vi "WLAN_be_EVM_SA_RS_CMP180.vi"(6 "SG Power":i32=-10, 7 "Function":T1, 8 "error in":errorcluster, 11 "VISA IN":refnum<visa-resource-name>="TCPIP0::192.168.200.50::hislip0::INSTR") -> (0 "error out":errorcluster, 1 "EVM":dbl format="%#.3g", 2 "Power":dbl format="%#.3g", 3 "IDN":string, 4 "FreqError":dbl)   [LabVIEW 2023, in "R_S.lvlib"]
uses:
  R_S.lvlib
  CTL/LitePoint_EVM_SA.ctl
panel:
  out "SecondTime":i32
  out "FirstTime":i32
  in  "Retry Times":i32=100
  out "Response":string
  out "String":string
  out "EVM_ALL_Carrier_Mean":string
  out "PPDU_Power_Mean":string
  out "VSA?":string
  # "CMP180: TCPIP0::192.168.200.50::hislip0::INSTR"
  # "TCPIP::Vince_Wu-NB::inst0::INSTR"
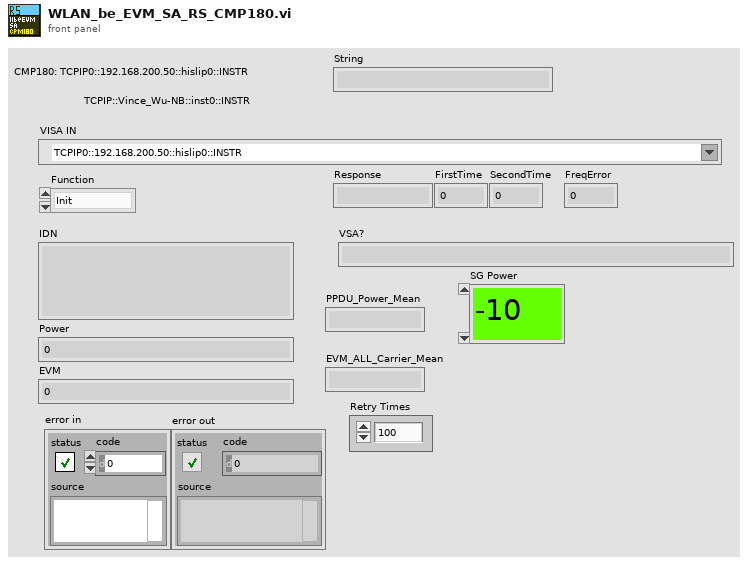
[diagram p1: front panel]
types:
  T1 = typedef "LitePoint_EVM_SA.ctl" = enum16{"Init", "Close", "set_SA", "get_EVM", "byPass", "getPower"}
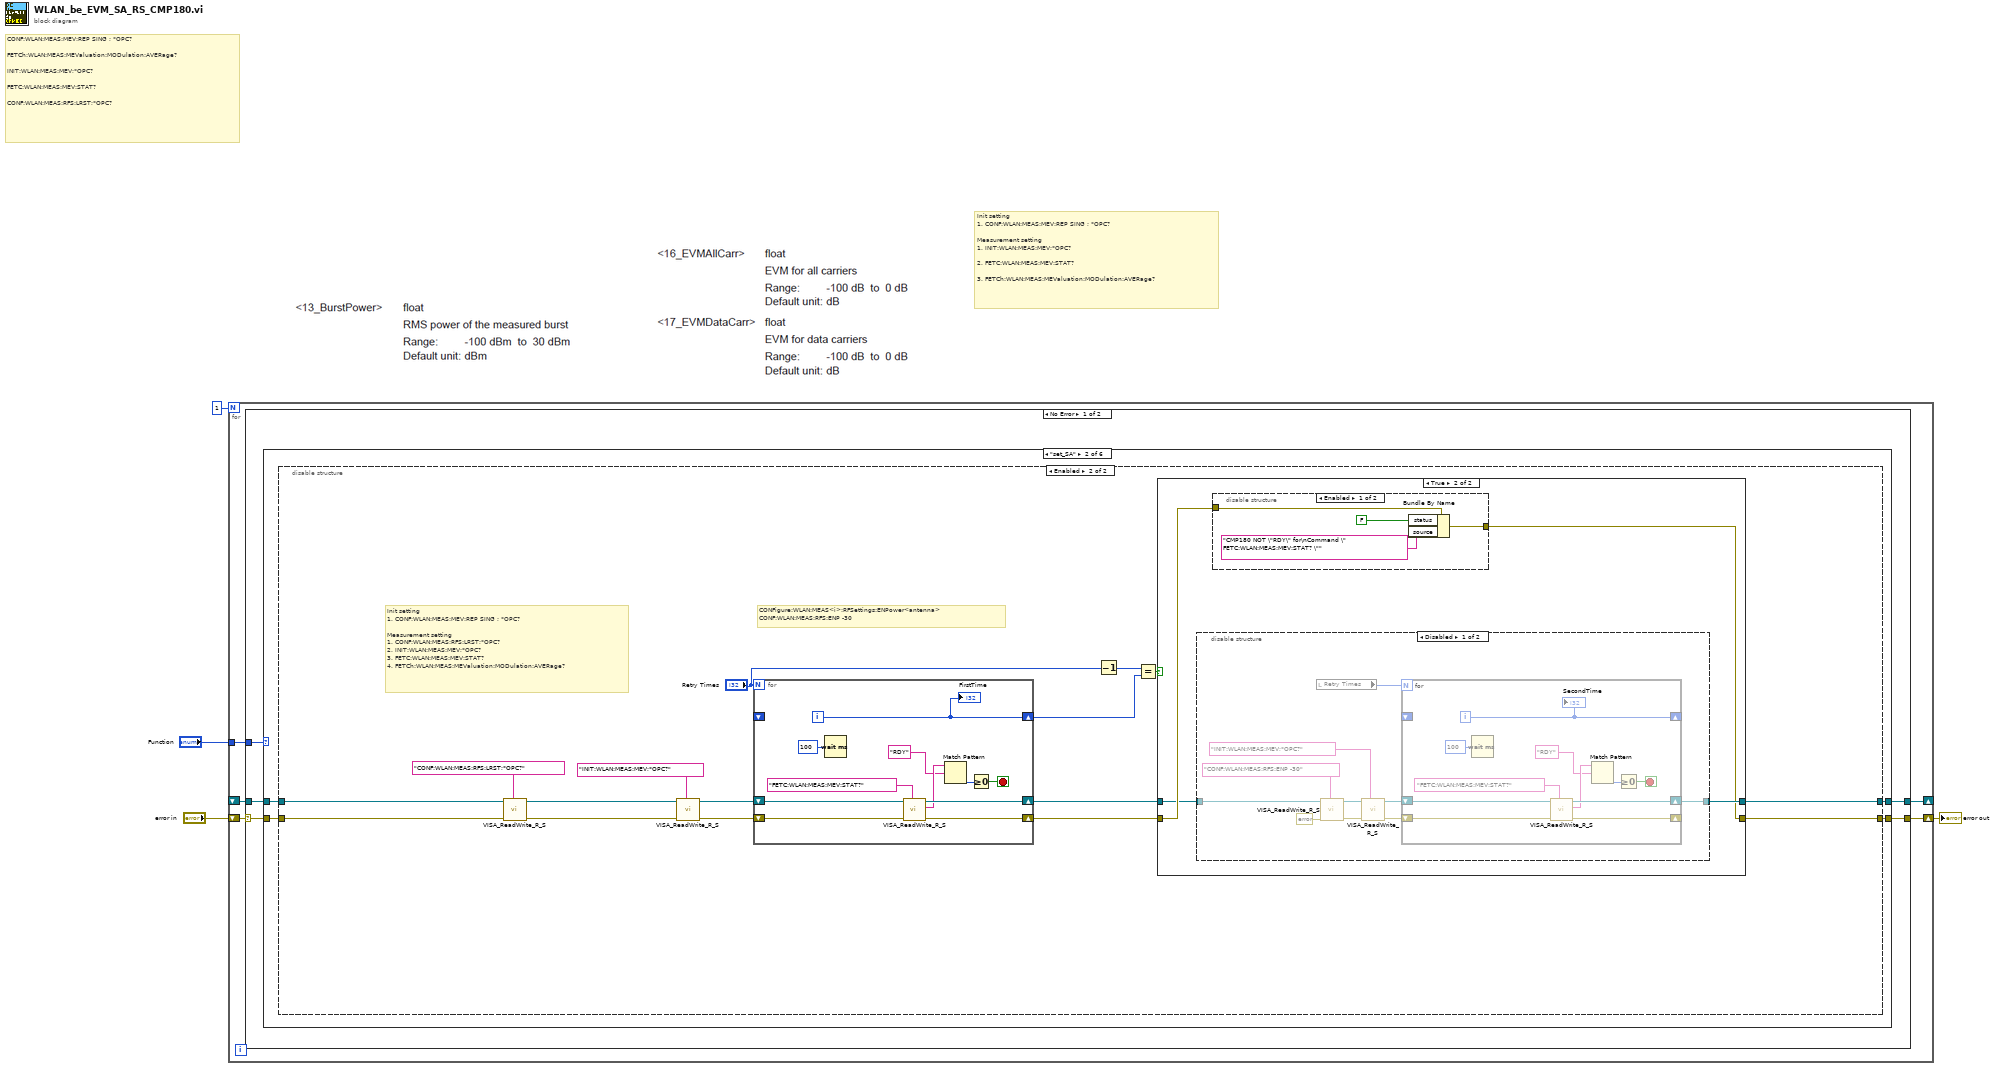
[diagram p0: block diagram]
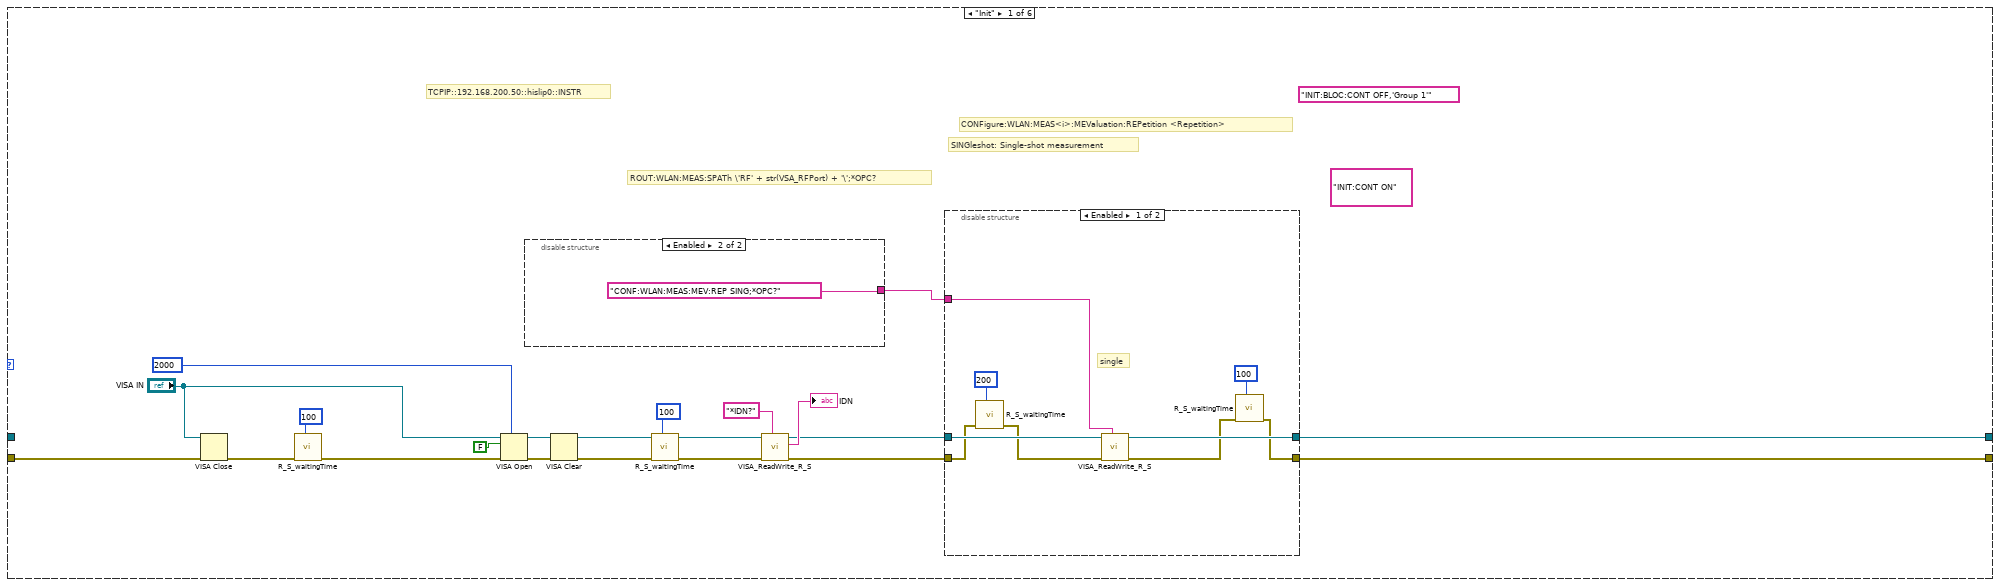
[diagram p2: hidden frame]
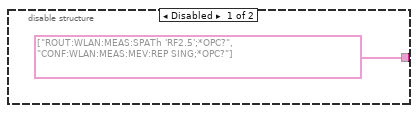
[diagram p3: hidden frame]
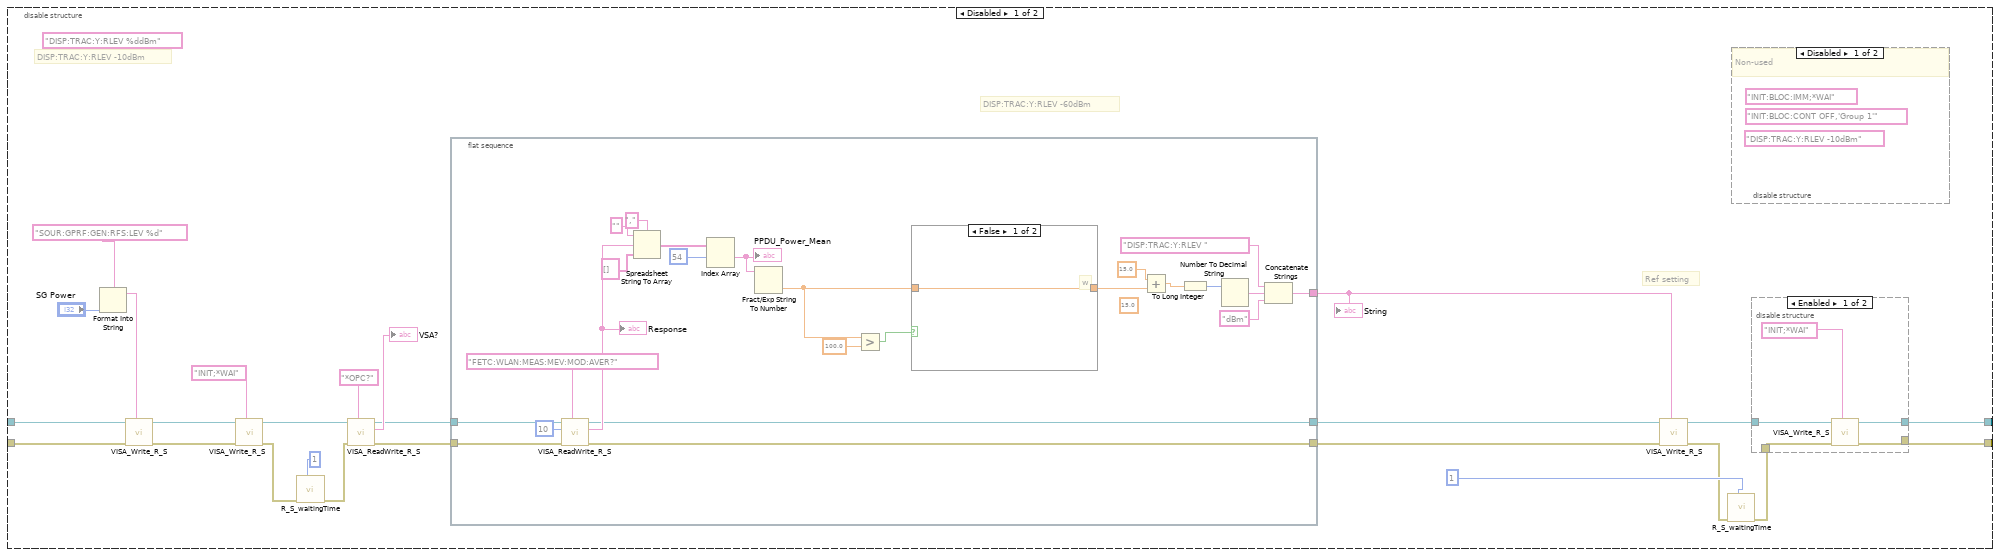
[diagram p5: hidden frame]
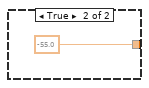
[diagram p7: hidden frame]
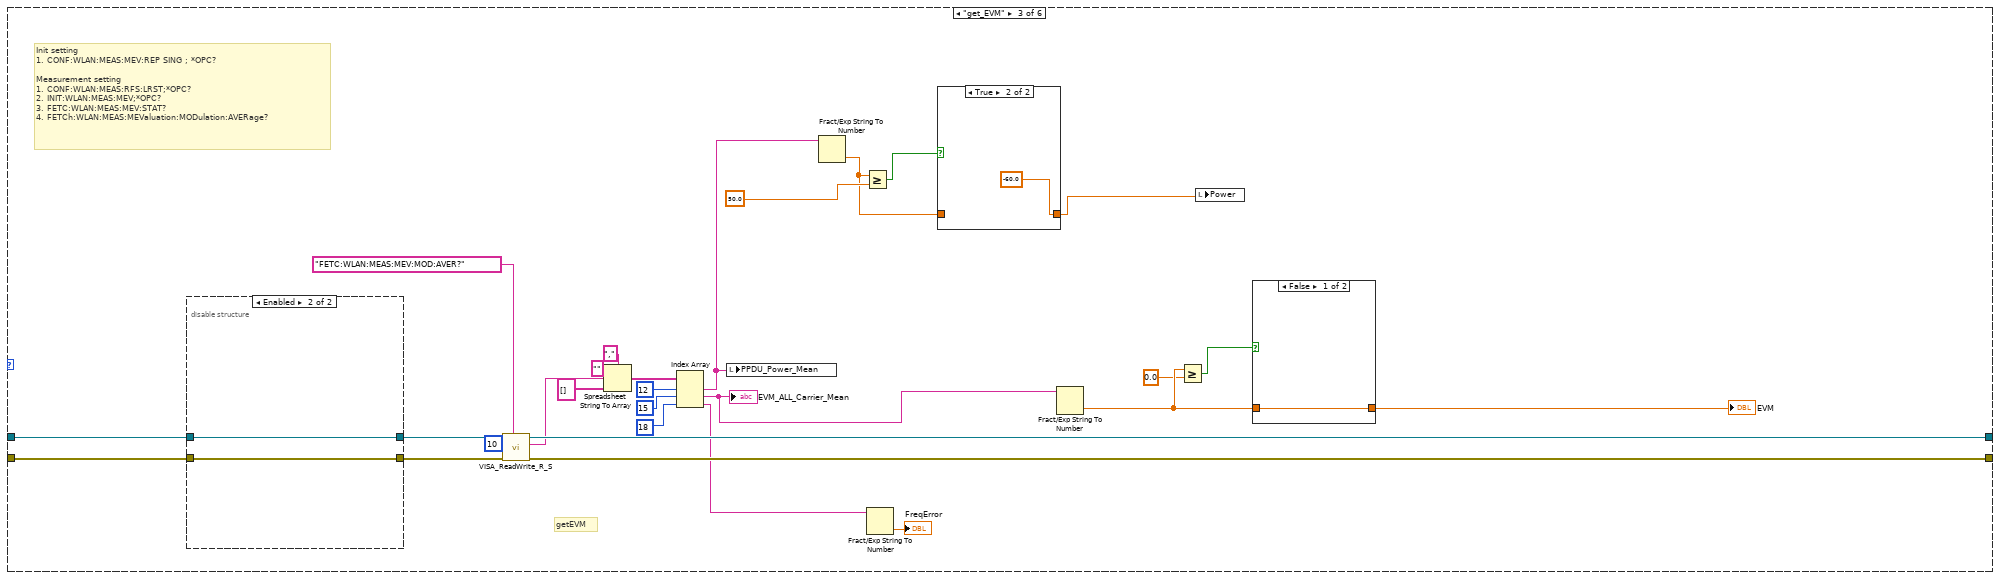
[diagram p12: hidden frame]
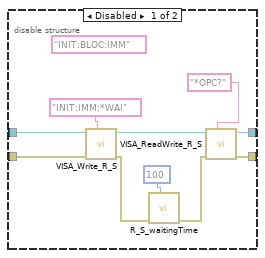
[diagram p13: hidden frame]
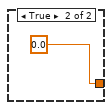
[diagram p15: hidden frame]
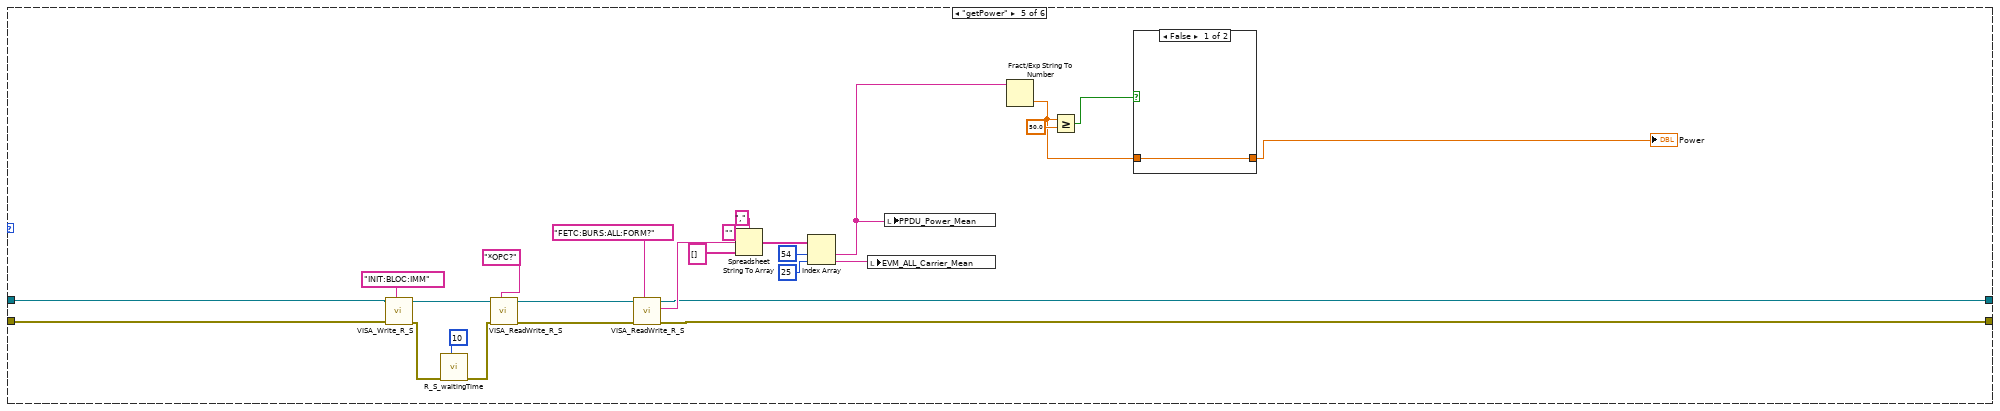
[diagram p17: hidden frame]
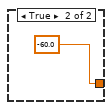
[diagram p18: hidden frame]
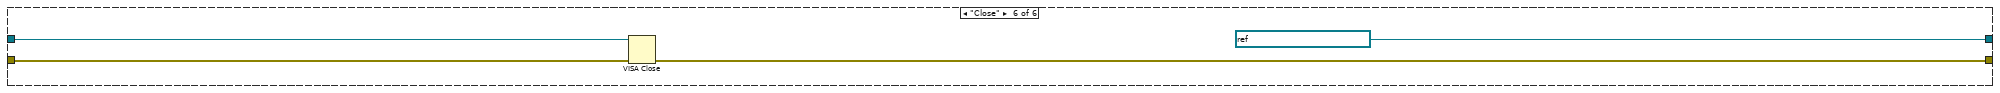
[diagram p19: hidden frame]
diagram:
  # "Init setting\n1. CONF:WLAN:MEAS:MEV:REP SING ; *OPC?\n\nMeasurement setting\n1. INIT:WLAN:MEAS:MEV;*OPC?\n\n2. FETC:WLAN:MEAS:MEV:STAT?\n\n3. FETCh:WLAN:MEAS:MEValuation:MODulation:AVERage?"
  # "CONF:WLAN:MEAS:MEV:REP SING ; *OPC?\n\nFETCh:WLAN:MEAS:MEValuation:MODulation:AVERage?\n\nINIT:WLAN:MEAS:MEV;*OPC?\n\nFETC:WLAN:MEAS:MEV:STAT?\n\nCONF:WLAN:MEAS:RFS:LRST;*OPC?"
  n1 = for {
    N: 1 -> [_]
    tunnel: "Function" -> [w7]
    shift-right: [w8] -> w3
    shift-left: "error in" -> [w9]
    shift-right: [w5] -> _
    shift-left: _ -> [w6]
    n2 = case shown="No Error" w9 {
      selector: w9 -> [w13 w249]
      tunnel: [w12 w249] -> w8
      tunnel: w7 -> [w14 _]
      tunnel: w6 -> [w11 w248]
      tunnel: [w10 w248] -> w5
      frame No Error {
        n3 = case shown="\"set_SA\"" w14 {
          tunnel: [w24 w51 w189 w215 w219 w247] -> w12
          tunnel: w13 -> [w27 w49 w190 w215 w221 w246]
          tunnel: w11 -> [_ w48 w188 w214 w222 w245]
          tunnel: [w22 w50 w187 w214 w220 refnum<visa-resource-name> refnum ("VISA out")] -> w10
          frame "Init" {
            (unwired) "INIT:BLOC:CONT OFF,'Group 1'"
            (unwired) "INIT:CONT ON"
            # "ROUT:WLAN:MEAS:SPATh \\'RF' + str(VSA_RFPort) + '\\';*OPC?"
            # "TCPIP::192.168.200.50::hislip0::INSTR"
            # "SINGleshot: Single-shot measurement"
            # "CONFigure:WLAN:MEAS<i>:MEValuation:REPetition <Repetition>"
            n4 = VISA Close(VISA resource name="VISA IN", error in (no error)=w27) -> (error out=w21:errorcluster)
            n5 = call "R_S_waitingTime.vi"("Waiting Time(ms)"=u32 100, "error in"=w21) -> ("error out"=w20:errorcluster)  [unwired: 9 in]
            n6 = VISA Open(timeout (0)=u32 2000 ("VISA Open timeout (0)"), duplicate session (F)=FALSE, error in (no error)=w20, VISA resource name="VISA IN") -> (VISA resource name=w31:refnum<visa-resource-name>, error out=w32:errorcluster)  [unwired: 1 in]
            n7 = disable-structure shown="Enabled" {
              disable-tunnel: [string[] ["ROUT:WLAN:MEAS:SPATh 'RF2.5';*OPC?", "CONF:WLAN:MEAS:MEV:REP SING;*OPC?"] "CONF:WLAN:MEAS:MEV:REP SING;*OPC?"] -> w15
              frame Disabled {
              }
              frame Enabled {
              }
            }
            n8 = VISA Clear(VISA resource name=w31, error in (no error)=w32) -> (VISA resource name out=w30:refnum<visa-resource-name>, error out=w17:errorcluster)
            n9 = call "R_S_waitingTime.vi"("Waiting Time(ms)"=u32 100, "error in"=w17) -> ("error out"=w16:errorcluster)  [unwired: 9 in]
            n10 = call "VISA_ReadWrite_R_S.vi"("VISA_CMD"="*IDN?", "error in"=w16, "VISA in"=w30) -> ("error out"=w25:errorcluster, "Response"=→"IDN":string, "VISA out"=w23:refnum<visa-resource-name>)  [unwired: 6 in]
            n11 = disable-structure shown="Enabled" {
              disable-tunnel: w25 -> [w41 w47]
              disable-tunnel: [w38 w47] -> w24
              disable-tunnel: w23 -> [w45 w46]
              disable-tunnel: [w44 w46] -> w22
              disable-tunnel: w15 -> [w37 _]
              frame Enabled {
                # "single"
                n12 = call "R_S_waitingTime.vi"("Waiting Time(ms)"=u32 200, "error in"=w41) -> ("error out"=w42:errorcluster)  [unwired: 9 in]
                n13 = call "VISA_ReadWrite_R_S.vi"("VISA_CMD"=w37, "error in"=w42, "VISA in"=w45) -> ("error out"=w39:errorcluster, "VISA out"=w44:refnum<visa-resource-name>)  [unwired: 6 in, 1 out]
                n14 = call "R_S_waitingTime.vi"("Waiting Time(ms)"=u32 100, "error in"=w39) -> ("error out"=w38:errorcluster)  [unwired: 9 in]
              }
              frame Disabled {
              }
            }
          }
          frame "set_SA" {
            n15 = disable-structure shown="Enabled" {
              disable-tunnel: [w63 w117] -> w51
              disable-tunnel: [w62 w115] -> w50
              disable-tunnel: w49 -> [w59 w111]
              disable-tunnel: w48 -> [w58 w110]
              frame Disabled {
                (unwired) "DISP:TRAC:Y:RLEV %ddBm" ("VISA CMD")
                # "DISP:TRAC:Y:RLEV -10dBm"
                # "Ref setting"
                # "DISP:TRAC:Y:RLEV -60dBm"
                n16 = Format Into String(format string="SOUR:GPRF:GEN:RFS:LEV %d" ("VISA CMD"), "SG Power") -> (resulting string=w52:string)  [unwired: 2 in, 1 out]
                n17 = call "VISA_Write_R_S.vi"("VISA CMD"=w52, "error in"=w59, "VISA in"=w58) -> ("error out"=w55:errorcluster, "VISA out"=w56:refnum<visa-resource-name>)  [unwired: 7 in]
                n18 = call "VISA_Write_R_S.vi"("VISA CMD"="INIT;*WAI", "error in"=w55, "VISA in"=w56) -> ("error out"=w61:errorcluster, "VISA out"=w60:refnum<visa-resource-name>)  [unwired: 7 in]
                n19 = call "R_S_waitingTime.vi"("Waiting Time(ms)"=u32 1, "error in"=w61) -> ("error out"=w76:errorcluster)  [unwired: 9 in]
                n20 = call "VISA_ReadWrite_R_S.vi"("VISA_CMD"="*OPC?", "error in"=w76, "VISA in"=w60) -> ("error out"=w72:errorcluster, "Response"=→"VSA?":string, "VISA out"=w71:refnum<visa-resource-name>)  [unwired: 6 in]
                n21 = flat-sequence {
                  tunnel: w72 -> [w100]
                  tunnel: w71 -> [w99]
                  tunnel: [w97] -> w70
                  tunnel: [w96] -> w69
                  tunnel: [w95] -> w68
                  frame #0 {
                    (unwired) 15.0 ("x")
                    n22 = call "VISA_ReadWrite_R_S.vi"("VISA_CMD"="FETC:WLAN:MEAS:MEV:MOD:AVER?", "error in"=w100, "waiting(ms)"=u32 10, "VISA in"=w99) -> ("error out"=w97:errorcluster, "Response"=w98:string, "VISA out"=w95:refnum<visa-resource-name>)  [unwired: 5 in]
                    "Response" <- w98
                    n23 = Spreadsheet String To Array(delimiter (Tab)=",", format string="", spreadsheet string=w98, array type (2D Dbl)=string[] []) -> (array=w83:string[])
                    n24 = Index Array(array=w83, index #1=54 ("index")) -> (element #1=w79:string)  [unwired: 1 in, 1 out]
                    "PPDU_Power_Mean" <- w79
                    n25 = Fract/Exp String To Number(string=w79) -> (number=w87:dbl)  [unwired: 3 in, 1 out]
                    n26 = Greater?(x=w87, y=100.0) -> (0:w85:bool)
                    n27 = case shown="False" w85 {
                      tunnel: w87 -> [w101 _]
                      tunnel: [w101 -55.0 ("y")] -> w88
                      frame False {
                        # "w"
                      }
                      frame True {
                      }
                    }
                    n28 = Add(x=15.0, y=w88) -> (x+y=w89:dbl)
                    n29 = To Long Integer(number=w89) -> (32bit integer=w78:i32)
                    n30 = Number To Decimal String(number=w78) -> (decimal integer string=w91:string)  [unwired: 1 in]
                    n31 = Concatenate Strings("DISP:TRAC:Y:RLEV " ("write buffer"), w91, "dBm" ("write buffer")) -> (w96:string)
                  }
                }
                n32 = call "VISA_Write_R_S.vi"("VISA CMD"=w69, "error in"=w70, "VISA in"=w68) -> ("error out"=w66:errorcluster, "VISA out"=w65:refnum<visa-resource-name>)  [unwired: 7 in]
                n33 = call "R_S_waitingTime.vi"("Waiting Time(ms)"=u32 1, "error in"=w66) -> ("error out"=w64:errorcluster)  [unwired: 9 in]
                n34 = disable-structure shown="Disabled" {
                  frame Disabled {
                    (unwired) "DISP:TRAC:Y:RLEV -10dBm" ("VISA CMD")
                    (unwired) "INIT:BLOC:IMM;*WAI"
                    (unwired) "INIT:BLOC:CONT OFF,'Group 1'"
                    # "Non-used"
                  }
                  frame Enabled {
                  }
                }
                n35 = disable-structure shown="Enabled" {
                  disable-tunnel: w65 -> [w107 w108]
                  disable-tunnel: w64 -> [w106 w109]
                  disable-tunnel: [w105 w109] -> w63
                  disable-tunnel: [w104 w108] -> w62
                  frame Enabled {
                    n36 = call "VISA_Write_R_S.vi"("VISA CMD"="INIT;*WAI", "error in"=w106, "VISA in"=w107) -> ("error out"=w105:errorcluster, "VISA out"=w104:refnum<visa-resource-name>)  [unwired: 7 in]
                  }
                  frame Disabled {
                  }
                }
                "String" <- w69
              }
              frame Enabled {
                # "CONFigure:WLAN:MEAS<i>:RFSettings:ENPower<antenna>\nCONF:WLAN:MEAS:RFS:ENP -30"
                # "Init setting\n1. CONF:WLAN:MEAS:MEV:REP SING ; *OPC?\n\nMeasurement setting\n1. CONF:WLAN:MEAS:RFS:LRST;*OPC?\n2. INIT:WLAN:MEAS:MEV;*OPC?\n3. FETC:WLAN:MEAS:MEV:STAT?\n4. FETCh:WLAN:MEAS:MEValuation:MODulation:AVERage?"
                n37 = call "VISA_ReadWrite_R_S.vi"("VISA_CMD"="CONF:WLAN:MEAS:RFS:LRST;*OPC?", "error in"=w111, "VISA in"=w110) -> ("error out"=w112:errorcluster, "VISA out"=w113:refnum<visa-resource-name>)  [unwired: 6 in, 1 out]
                n38 = call "VISA_ReadWrite_R_S.vi"("VISA_CMD"="INIT:WLAN:MEAS:MEV;*OPC?", "error in"=w112, "VISA in"=w113) -> ("error out"=w124:errorcluster, "VISA out"=w123:refnum<visa-resource-name>)  [unwired: 6 in, 1 out]
                n39 = for {
                  N: "Retry Times" -> [_]
                  shift-right: [w165] -> w116
                  shift-left: w123 -> [w168]
                  shift-right: [w166] -> w118
                  shift-left: w124 -> [w169]
                  shift-right: [w160] -> w121
                  shift-left: _ -> [_]
                  i -> [w160]
                  stop <- w161 stop-if-true
                  n40 = Wait (ms)(milliseconds to wait=u32 100) -> ()  [unwired: 1 out]
                  n41 = call "VISA_ReadWrite_R_S.vi"("VISA_CMD"="FETC:WLAN:MEAS:MEV:STAT?", "error in"=w169, "VISA in"=w168) -> ("error out"=w166:errorcluster, "Response"=w164:string, "VISA out"=w165:refnum<visa-resource-name>)  [unwired: 6 in]
                  n42 = Match Pattern(string=w164, regular expression="RDY") -> (offset past match=w162:i32)  [unwired: 1 in, 3 out]
                  n43 = Greater Or Equal To 0?(x=w162) -> (x >= 0?=w161:bool)
                  "FirstTime" <- w160
                }
                n44 = Decrement(x="Retry Times") -> (x-1=w120:i32)
                n45 = Equal?(x=w120, y=w121) -> (x = y?=w119:bool)
                n46 = case shown="True" w119 {
                  tunnel: w118 -> [w127 w131]
                  tunnel: [w127 w128] -> w117
                  tunnel: w116 -> [w126 w130]
                  tunnel: [w126 w129] -> w115
                  frame False {
                  }
                  frame True {
                    n47 = disable-structure shown="Disabled" {
                      disable-tunnel: w130 -> [w140 w153]
                      disable-tunnel: [w133 w153] -> w129
                      frame Disabled {
                        n48 = local read "Retry Times"() -> (w136:i32)
                        n49 = call "VISA_ReadWrite_R_S.vi"("VISA_CMD"="CONF:WLAN:MEAS:RFS:ENP -30", "error in"=errorcluster {"status"=FALSE, "code"=0, "source"=""}, "VISA in"=w140) -> ("error out"=w139:errorcluster, "VISA out"=w135:refnum<visa-resource-name>)  [unwired: 6 in, 1 out]
                        n50 = call "VISA_ReadWrite_R_S.vi"("VISA_CMD"="INIT:WLAN:MEAS:MEV;*OPC?", "error in"=w139, "VISA in"=w135) -> ("error out"=w137:errorcluster, "VISA out"=w134:refnum<visa-resource-name>)  [unwired: 6 in, 1 out]
                        n51 = for {
                          N: w136 -> [_]
                          shift-right: [w148] -> w133
                          shift-left: w134 -> [w151]
                          shift-right: [w149] -> _
                          shift-left: w137 -> [w152]
                          shift-right: [w143] -> _
                          shift-left: _ -> [_]
                          i -> [w143]
                          stop <- w144 stop-if-true
                          n52 = Wait (ms)(milliseconds to wait=u32 100) -> ()  [unwired: 1 out]
                          n53 = call "VISA_ReadWrite_R_S.vi"("VISA_CMD"="FETC:WLAN:MEAS:MEV:STAT?", "error in"=w152, "VISA in"=w151) -> ("error out"=w149:errorcluster, "Response"=w147:string, "VISA out"=w148:refnum<visa-resource-name>)  [unwired: 6 in]
                          n54 = Match Pattern(string=w147, regular expression="RDY") -> (offset past match=w145:i32)  [unwired: 1 in, 3 out]
                          n55 = Greater Or Equal To 0?(x=w145) -> (x >= 0?=w144:bool)
                          "SecondTime" <- w143
                        }
                      }
                      frame Enabled {
                      }
                    }
                    n56 = disable-structure shown="Enabled" {
                      disable-tunnel: w131 -> [w155 w158]
                      disable-tunnel: [w154 w158] -> w128
                      frame Enabled {
                        n57 = Bundle By Name(cluster=w155, "status"=FALSE, "source"="CMP180 NOT \"RDY\" for\nCommand \" FETC:WLAN:MEAS:MEV:STAT? \"") -> (w154:errorcluster)
                      }
                      frame Disabled {
                      }
                    }
                  }
                }
              }
            }
          }
          frame "get_EVM" {
            # "Init setting\n1. CONF:WLAN:MEAS:MEV:REP SING ; *OPC?\n\nMeasurement setting\n1. CONF:WLAN:MEAS:RFS:LRST;*OPC?\n2. INIT:WLAN:MEAS:MEV;*OPC?\n3. FETC:WLAN:MEAS:MEV:STAT?\n4. FETCh:WLAN:MEAS:MEValuation:MODulation:AVERage?"
            # "getEVM"
            n58 = disable-structure shown="Enabled" {
              disable-tunnel: [w204 w209] -> w193
              disable-tunnel: [w203 w208] -> w192
              disable-tunnel: w190 -> [w199 w209]
              disable-tunnel: w188 -> [w198 w208]
              frame Disabled {
                (unwired) "INIT:BLOC:IMM"
                n59 = call "VISA_Write_R_S.vi"("VISA CMD"="INIT:IMM;*WAI", "error in"=w199, "VISA in"=w198) -> ("error out"=w206:errorcluster, "VISA out"=w207:refnum<visa-resource-name>)  [unwired: 7 in]
                n60 = call "R_S_waitingTime.vi"("Waiting Time(ms)"=u32 100, "error in"=w206) -> ("error out"=w205:errorcluster)  [unwired: 9 in]
                n61 = call "VISA_ReadWrite_R_S.vi"("VISA_CMD"="*OPC?", "error in"=w205, "VISA in"=w207) -> ("error out"=w204:errorcluster, "VISA out"=w203:refnum<visa-resource-name>)  [unwired: 6 in, 1 out]
              }
              frame Enabled {
              }
            }
            n62 = call "VISA_ReadWrite_R_S.vi"("VISA_CMD"="FETC:WLAN:MEAS:MEV:MOD:AVER?", "error in"=w193, "waiting(ms)"=u32 10, "VISA in"=w192) -> ("error out"=w189:errorcluster, "Response"=w180:string, "VISA out"=w187:refnum<visa-resource-name>)  [unwired: 5 in]
            n63 = Spreadsheet String To Array(delimiter (Tab)=",", format string="", spreadsheet string=w180, array type (2D Dbl)=string[] []) -> (array=w184:string[])
            n64 = Index Array(array=w184, index #1=12 ("index"), index #2=15 ("index"), index #3=18 ("index")) -> (element #1=w175:string, element #2=w179:string, element #3=w171:string)
            "EVM_ALL_Carrier_Mean" <- w179
            n65 = local write "PPDU_Power_Mean"(w175) -> ()
            n66 = Fract/Exp String To Number(string=w175) -> (number=w176:dbl)  [unwired: 3 in, 1 out]
            n67 = Greater Or Equal?(x=w176, y=50.0) -> (x >= y?=w177:bool)
            n68 = Fract/Exp String To Number(string=w171) -> (number=→"FreqError":dbl)  [unwired: 3 in, 1 out]
            n69 = case shown="True" w177 {
              tunnel: w176 -> [w210 _]
              tunnel: [w210 -60.0] -> w174
              frame False {
              }
              frame True {
              }
            }
            n70 = Fract/Exp String To Number(string=w179) -> (number=w196:dbl)  [unwired: 3 in, 1 out]
            n71 = Greater Or Equal?(x=w196, y=0.0) -> (x >= y?=w194:bool)
            n72 = local write "Power"(w174) -> ()
            n73 = case shown="False" w194 {
              tunnel: w196 -> [w212 _]
              tunnel: [w212 0.0] -> w197
              frame False {
              }
              frame True {
              }
            }
            "EVM" <- w197
          }
          frame "byPass", Default {
          }
          frame "getPower" {
            n74 = call "VISA_Write_R_S.vi"("VISA CMD"="INIT:BLOC:IMM", "error in"=w221, "VISA in"=w222) -> ("error out"=w236:errorcluster, "VISA out"=w237:refnum<visa-resource-name>)  [unwired: 7 in]
            n75 = call "R_S_waitingTime.vi"("Waiting Time(ms)"=u32 10, "error in"=w236) -> ("error out"=w235:errorcluster)  [unwired: 9 in]
            n76 = call "VISA_ReadWrite_R_S.vi"("VISA_CMD"="*OPC?", "error in"=w235, "VISA in"=w237) -> ("error out"=w234:errorcluster, "VISA out"=w218:refnum<visa-resource-name>)  [unwired: 6 in, 1 out]
            n77 = call "VISA_ReadWrite_R_S.vi"("VISA_CMD"="FETC:BURS:ALL:FORM?", "error in"=w234, "VISA in"=w218) -> ("error out"=w219:errorcluster, "Response"=w223:string, "VISA out"=w220:refnum<visa-resource-name>)  [unwired: 6 in]
            n78 = Spreadsheet String To Array(delimiter (Tab)=",", format string="", spreadsheet string=w223, array type (2D Dbl)=string[] []) -> (array=w227:string[])
            n79 = Index Array(array=w227, index #1=54 ("index"), index #2=25 ("index")) -> (element #1=w216:string, element #2=w217:string)
            n80 = local write "EVM_ALL_Carrier_Mean"(w217) -> ()
            n81 = local write "PPDU_Power_Mean"(w216) -> ()
            n82 = Fract/Exp String To Number(string=w216) -> (number=w239:dbl)  [unwired: 3 in, 1 out]
            n83 = Greater Or Equal?(x=w239, y=50.0) -> (x >= y?=w240:bool)
            n84 = case shown="False" w240 {
              tunnel: w239 -> [w242 _]
              tunnel: [w242 -60.0] -> w238
              frame False {
              }
              frame True {
              }
            }
            "Power" <- w238
          }
          frame "Close" {
            n85 = VISA Close(VISA resource name=w245, error in (no error)=w246) -> (error out=w247:errorcluster)
          }
        }
      }
      frame Error {
      }
    }
  }
  "error out" <- w3
